vi "ClimberBegin.vi"(8 "error in (no error)":errorcluster, 10 "Configuration In":variant, 11 "Climber in":refnum<class "Climber.lvclass">) -> (0 "error out":errorcluster, 3 "Climber out":refnum<class "Climber.lvclass">)   [LabVIEW 2019, in "Climber.lvlib" / "Climber.lvclass"]
uses:
  Climber.lvclass
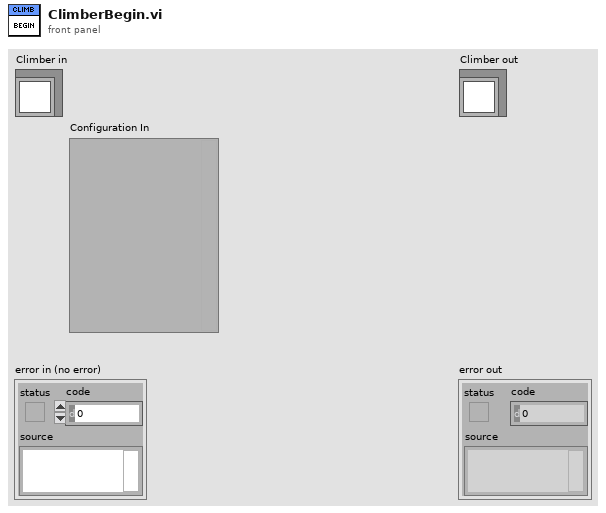
[diagram p1: front panel]
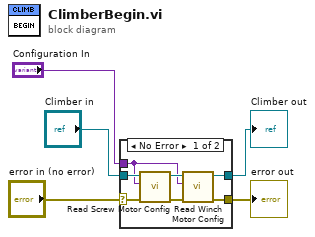
[diagram p0: block diagram]
diagram:
  n1 = case shown="No Error" "error in (no error)" {
    selector: "error in (no error)" -> [w9 w14]
    tunnel: [w7 w14] -> w4
    tunnel: [w10 w13] -> w2
    tunnel: "Climber in" -> [w12 w13]
    tunnel: "Configuration In" -> [w6 _]
    frame No Error {
      n2 = call "Read Screw Motor Config.vi"("error in (no error)"=w9, "Configuration In"=w6, "Climber in"=w12) -> ("error out"=w8:errorcluster, "Climber out"=w11:refnum<class "Climber.lvclass">)  [unwired: 7 in]
      n3 = call "Read Winch Motor Config.vi"("error in (no error)"=w8, "Configuration In"=w6, "Climber in"=w11) -> ("error out"=w7:errorcluster, "Climber out"=w10:refnum<class "Climber.lvclass">)  [unwired: 7 in]
    }
    frame Error {
    }
  }
  "error out" <- w4
  "Climber out" <- w2
